vi "ShooterState.vi"(10 "Set?":bool, 11 "Value in":T1=enum."Ready") -> (3 "Value out":T1=enum."Ready")   [LabVIEW 2013]
doc: "Functional Global to handle comunication of shooter state"
uses:
  ShooterStates.ctl
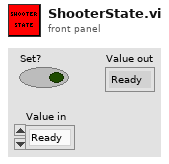
[diagram p1: front panel]
types:
  T1 = typedef "ShooterStates.ctl" = enum16{"Init", "Ready", "RetractFull", "Disengage Clutch", "Clutch Delay", "Fire", "Fire Delay", "Latch", "Retract", "Release"}
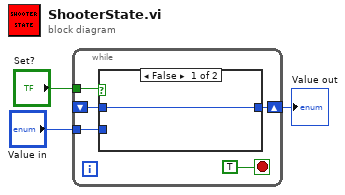
[diagram p0: block diagram]
diagram:
  n1 = while {
    tunnel: "Set?" -> [w8]
    tunnel: "Value in" -> [w7]
    shift-right: [w6] -> w3
    shift-left: _ -> [w5]
    stop <- TRUE stop-if-true
    n2 = case shown="False" w8 {
      tunnel: w7 -> [_ w10]
      tunnel: [w9 w10] -> w6
      tunnel: w5 -> [w9 _]
      frame False {
      }
      frame True {
      }
    }
  }
  "Value out" <- w3
